vi "f2.vi"() -> ()   [LabVIEW 2016]
uses:
  <vilib>/Utility/miscctls.llb/LVMouseTypeDef.ctl
panel:
  out "Waveform Graph 4":waveform(dbl)(graph)
  out "Mouse":T1
  in  "Stop Button":bool
  in  "pen":T2={"Width"=1, "Style"=enum."Solid"}
  out "new picture":picture
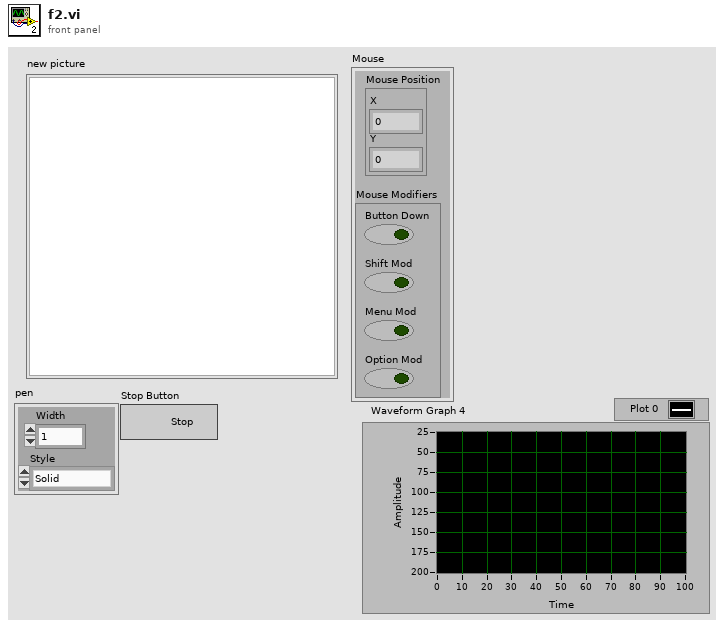
[diagram p1: front panel]
types:
  T1 = typedef "LVMouseTypeDef.ctl" = cluster{"Mouse Position":cluster{"X":i32, "Y":i32}, "Mouse Modifiers":cluster{"Button Down":bool, "Shift Mod":bool, "Menu Mod":bool, "Option Mod":bool}}
  T2 = cluster{"Width":u16, "Style":enum32{"Solid", "Dash", "Dot", "DashDot", "DashDotDot"}}
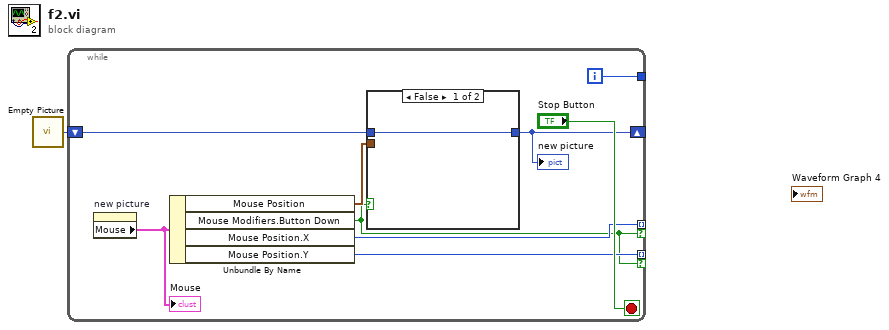
[diagram p0: block diagram]
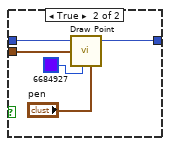
[diagram p2: hidden frame]
diagram:
  n1 = call "Empty Picture"() -> ("empty picture"=w1:picture)
  n2 = while {
    shift-right: [w9] -> _
    shift-left: w1 -> [w8]
    tunnel: [w5] -> _ mode=indexing if=w3
    tunnel: [w4] -> _ mode=indexing if=w3
    tunnel: [w2] -> _
    i -> [w2]
    stop <- "Stop Button" stop-if-true
    n3 = property on="new picture" class="Pict"() -> ("Mouse"=w7:T1)  [unwired: 2 in, 2 out]
    "Mouse" <- w7
    n4 = Unbundle By Name(w7) -> ("Mouse Position"=w6:cluster{"X":i32, "Y":i32}, "Mouse Modifiers.Button Down"=w3:bool, "Mouse Position.X"=w5:i32, "Mouse Position.Y"=w4:i32)
    n5 = case shown="False" w3 {
      tunnel: [w11 w14] -> w9
      tunnel: w8 -> [w11 w13]
      tunnel: w6 -> [_ w12]
      frame False {
      }
      frame True {
        n6 = call <vilib>:"Draw Point.vi"("picture"=w13, "point(x,y)"=w12, "color(black)"=u32 6684927, "pen"="pen") -> ("new picture"=w14:picture)  [unwired: 5 in]
      }
    }
    "new picture" <- w9
  }
